vi "Read Baud Rate.vi"(8 "error in (no error)":errorcluster, 11 "VGC in":refnum<class "PL Inficon VGC.lvclass">) -> (0 "error out":errorcluster, 2 "baud rate":u32(ring)=115200 items=["9600"=9600, "19200"=19200, "38400"=38400, "57600"=57600, "115200"=115200], 3 "VGC out":refnum<class "PL Inficon VGC.lvclass">)   [LabVIEW 2015, in "PL Inficon VGC.lvclass"]
doc: "Reads baud rate."
uses:
  PL Inficon VGC.lvclass
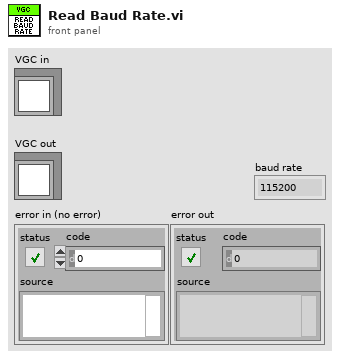
[diagram p1: front panel]
types:
  T1 = typedef "LVStringsAndValuesArrayTypeDef_U32.ctl" = cluster{"String":string, "Value":u32}[]
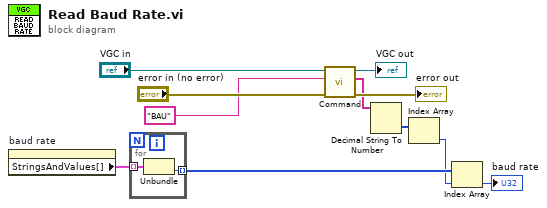
[diagram p0: block diagram]
diagram:
  n1 = property on="baud rate" class="Ring (strict)"() -> ("StringsAndValues[]"=w4:T1)  [unwired: 2 in, 2 out]
  n2 = for {
    tunnel: w4 -> [w13] mode=indexing
    tunnel: [w12] -> w3 mode=indexing
    n3 = Unbundle(w13) -> ("Value"=w12:u32)  [unwired: 1 out]
  }
  n4 = call "Command.vi"("error in (no error)"="error in (no error)", "command"="BAU" ("format string"), "VGC in"="VGC in") -> ("error out"=→"error out":errorcluster, "response data"=w6:string[], "VGC out"=→"VGC out":refnum<class "PL Inficon VGC.lvclass">)  [unwired: 6 in]
  n5 = Decimal String To Number(string=w6) -> (number=w7:i32[])  [unwired: 2 in, 1 out]
  n6 = Index Array(array=w7) -> (element=w2:i32)  [unwired: 1 in]
  n7 = Index Array(array=w3, index=w2) -> (element=→"baud rate":u32)
